vi "K2602 setImeasV.vi"(8 "Settings":T1={"Channel"=enum."Channel A", "Vset"=1e-05, "NPLC"=1.0, "I compliance"=3.0, "Repeat time"=3, "Delay ms"=10.0, "4-wire"=FALSE}, 11 "SMU":refnum<visa-resource-name>="GPIB0::26::INSTR") -> (0 "error out":errorcluster, 1 "Vavg":dbl=0.09425289999999999, 2 "Imeas":dbl[](array[numeric])=[1e-05, 1e-05, 1e-05], 3 "Vmeas":dbl[](array[numeric])=[0.0943061, 0.0942282, 0.0942244])   [LabVIEW 2012]
uses:
  SMU Settings.ctl
  <instrlib>/KE26XX/KE26XX.lvlib
  <vilib>/Analysis/NI_AALBase.lvlib
panel:
  out "Final Script":string="smu = smua\r\nsmusense = smu.SENSE_LOCAL\r\niset = 1.000000E-5\r\nnplc = 1.000000E+0\r\nvlimit = 3.000000E+0\r\nreptime = 3\r\ndelaytime = 1.000000E-2\r\nsmu.reset()\nsmu.source.func = smu.OUTPUT_DCAMPS\nsmu.measure.autozero\t= smu.AUTOZERO_ONCE\nsmu.measure.autorangev\t= smu.AUTORANGE_ON\nsmu.source.autorangei\t= smu.AUTORANGE_ON\nsmu.sense = smusense\n\nsmu.source.leveli = iset\nsmu.source.limitv = vlimit\nsmu.measure.nplc = nplc \n\n-- Setup a buffer to store the result(s) in and start testing.\nsmu.nvbuffer1.clear()\nsmu.nvbuffer1.appendmode = 1\nsmu.nvbuffer1.collecttimestamps = 1\nsmu.nvbuffer1.collectsourcevalues = 1\nsmu.source.output = smu.OUTPUT_ON\n\nfor j = 1,reptime do\n    smu.source.leveli = iset\n    if j == 1 then\n        delay(0.01)  \n    end\n\t   delay(delaytime)                  -- Wait desired settling time.\n    smu.measure.v(smu.nvbuffer1)  -- Measure voltage and store in reading buffer.\nend\nsmu.source.output = smu.OUTPUT_OFF"
  in  "Vmeas Script":string="smu.reset()\nsmu.source.func = smu.OUTPUT_DCAMPS\nsmu.measure.autozero\t= smu.AUTOZERO_ONCE\nsmu.measure.autorangev\t= smu.AUTORANGE_ON\nsmu.source.autorangei\t= smu.AUTORANGE_ON\nsmu.sense = smusense\n\nsmu.source.leveli = iset\nsmu.source.limitv = vlimit\nsmu.measure.nplc = nplc \n\n-- Setup a buffer to store the result(s) in and start testing.\nsmu.nvbuffer1.clear()\nsmu.nvbuffer1.appendmode = 1\nsmu.nvbuffer1.collecttimestamps = 1\nsmu.nvbuffer1.collectsourcevalues = 1\nsmu.source.output = smu.OUTPUT_ON\n\nfor j = 1,reptime do\n    smu.source.leveli = iset\n    if j == 1 then\n        delay(0.01)  \n    end\n\t   delay(delaytime)                  -- Wait desired settling time.\n    smu.measure.v(smu.nvbuffer1)  -- Measure voltage and store in reading buffer.\nend\nsmu.source.output = smu.OUTPUT_OFF"
  in  "Read Points":u32=50
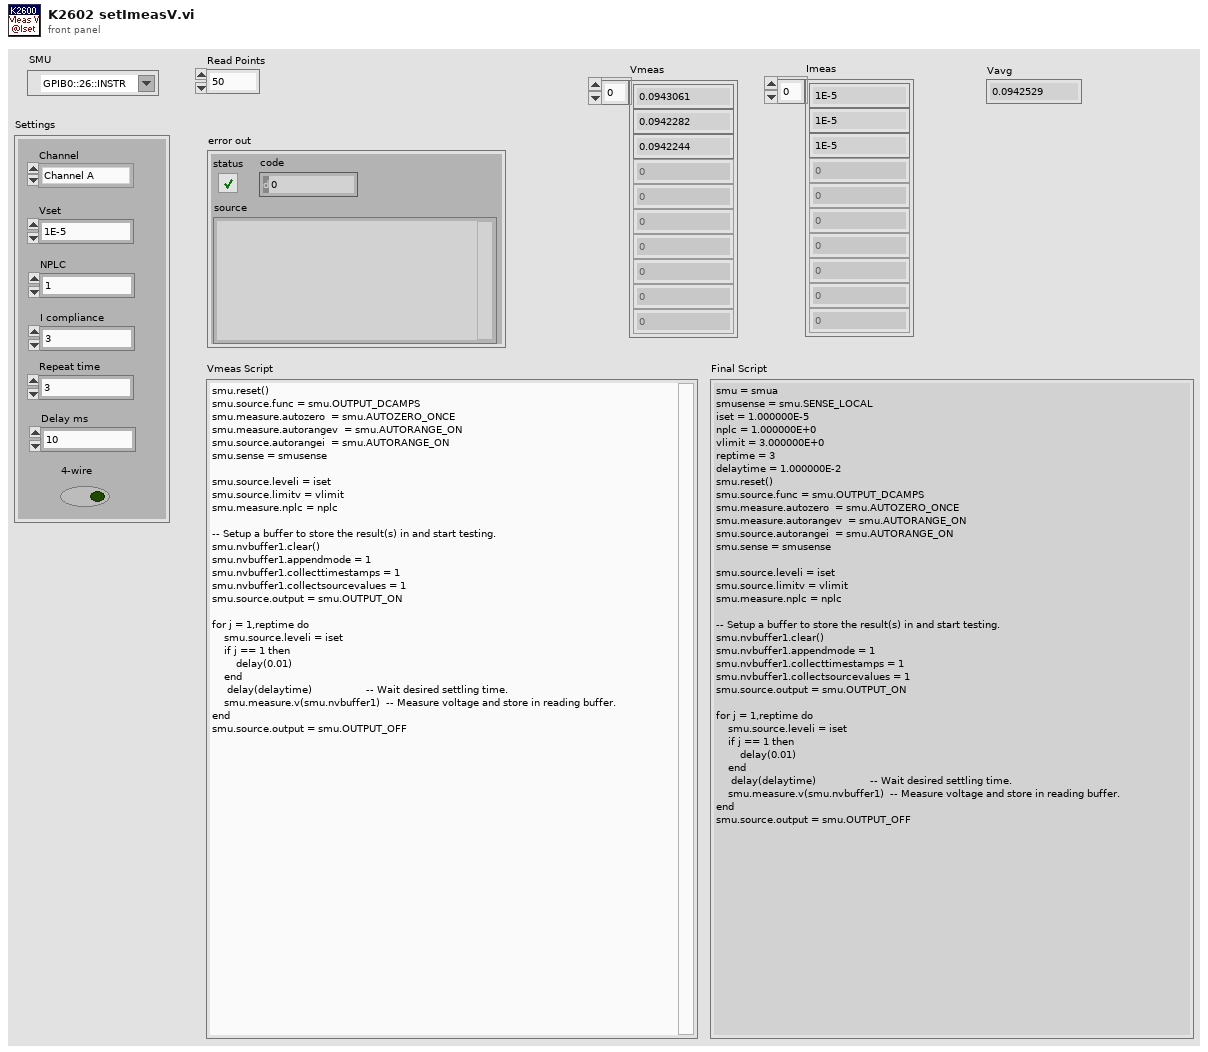
[diagram p1: front panel]
types:
  T1 = typedef "SMU Settings.ctl" = cluster{"Channel":enum32{"Channel A", "Channel B"}, "Vset":dbl, "NPLC":dbl, "I compliance":dbl, "Repeat time":u16, "Delay ms":dbl, "4-wire":bool}
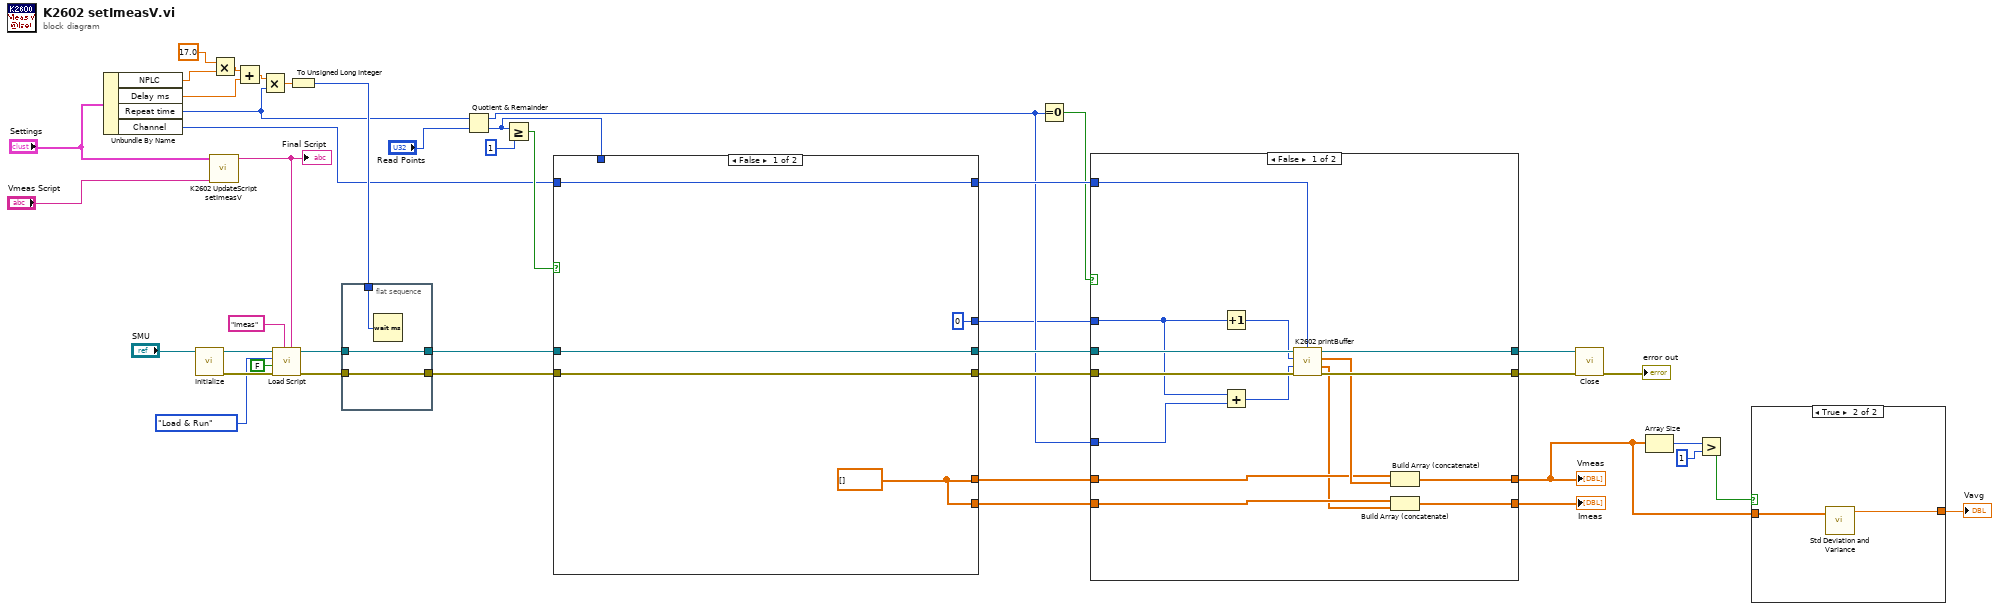
[diagram p0: block diagram]
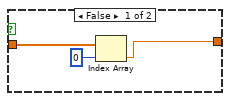
[diagram p2: hidden frame]
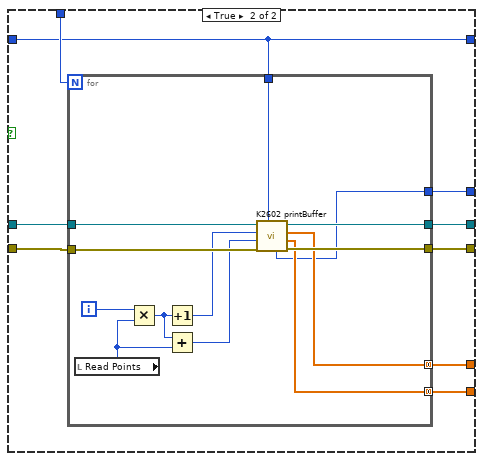
[diagram p4: hidden frame]
diagram:
  n1 = Unbundle By Name("Settings") -> ("NPLC"=w35:dbl, "Delay ms"=w4:dbl, "Repeat time"=w2:u16, "Channel"=w26:enum32{"Channel A", "Channel B"})
  n2 = call <instrlib>:"Initialize.vi"("VISA resource name"="SMU") -> ("error out"=w41:errorcluster, "VISA resource name out"=w42:refnum<visa-resource-name>)  [unwired: 9 in]
  n3 = call "K2602 UpdateScript setImeasV.vi"("Script"="Vmeas Script", "Settings"="Settings") -> ("Output"=w32:string)  [unwired: 9 in]
  "Final Script" <- w32
  n4 = Multiply(x=17.0, y=w35) -> (x*y=w5:dbl)
  n5 = Add(x=w5, y=w4) -> (x+y=w3:dbl)
  n6 = Multiply(x=w3, y=w2) -> (x*y=w1:dbl)
  n7 = call <instrlib>:"Load Script.vi"("Script"=w32, "Script Name"="Imeas", "error in"=w41, "Save (No)"=FALSE, "Load Options (Load)"=enum16{"Load", "Load & Run"}."Load & Run", "VISA resource name"=w42) -> ("error out"=w30:errorcluster, "VISA resource name out"=w31:refnum<visa-resource-name>)  [unwired: 4 out]
  n8 = To Unsigned Long Integer(number=w1) -> (unsigned 32bit integer=w33:u32)
  n9 = flat-sequence {
    tunnel: w33 -> [w46]
    tunnel: w31 -> [w45]
    tunnel: [w45] -> w24
    tunnel: w30 -> [w44]
    tunnel: [w44] -> w23
    frame #0 {
      n10 = Wait (ms)(milliseconds to wait=w46) -> ()  [unwired: 1 out]
    }
  }
  n11 = Quotient & Remainder(x=w2, y="Read Points") -> (x-y*floor(x/y)=w13:u32, floor(x/y)=w25:u32)
  n12 = Greater Or Equal?(x=w25, y=u32 1) -> (x >= y?=w27:bool)
  n13 = case shown="False" w27 {
    tunnel: w26 -> [w51 w55]
    tunnel: [w51 w55] -> w22
    tunnel: w25 -> [_ w60]
    tunnel: w24 -> [w50 w59]
    tunnel: w23 -> [w49 w58]
    tunnel: [w50 w57] -> w19
    tunnel: [w49 w56] -> w18
    tunnel: [w48 w54] -> w21
    tunnel: [w48 w53] -> w20
    tunnel: [u32 0 ("End Index out") w52] -> w11
    frame False {
      w48 = dbl[] [] ("array type (2D Dbl)")
    }
    frame True {
      n14 = for {
        N: w60 -> [_]
        tunnel: w59 -> [w73]
        tunnel: w58 -> [w72]
        tunnel: [w71] -> w57
        tunnel: [w70] -> w56
        tunnel: w55 -> [w69]
        tunnel: [w63] -> w54 mode=concatenating
        tunnel: [w62] -> w53 mode=concatenating
        tunnel: [w61] -> w52
        i -> [w68]
        n15 = local read "Read Points"() -> (w66:u32)
        n16 = Multiply(x=w68, y=w66) -> (x*y=w67:u32)
        n17 = Increment(x=w67) -> (x+1=w65:u32)
        n18 = Add(x=w67, y=w66) -> (x+y=w64:u32)
        n19 = call "K2602 printBuffer.vi"("Channel"=w69, "error in (no error)"=w72, "End Index"=w64, "Start Index"=w65, "SMU"=w73) -> ("error out"=w70:errorcluster, "V array"=w62:dbl[], "I array"=w63:dbl[], "SMU out"=w71:refnum<visa-resource-name>, "End Index out"=w61:u32)  [unwired: 2 in]
      }
    }
  }
  n20 = Equal To 0?(x=w13) -> (x = 0?=w12:bool)
  n21 = case shown="False" w12 {
    tunnel: w22 -> [w84 _]
    tunnel: w21 -> [w78 w90]
    tunnel: w20 -> [w76 w89]
    tunnel: w19 -> [w88 w92]
    tunnel: w18 -> [w87 w91]
    tunnel: [w86 w92] -> w17
    tunnel: [w85 w91] -> w16
    tunnel: [w77 w90] -> w7
    tunnel: [w74 w89] -> w15
    tunnel: w13 -> [w81 _]
    tunnel: w11 -> [w82 _]
    frame False {
      n22 = Increment(x=w82) -> (x+1=w83:u32)
      n23 = Add(x=w82, y=w81) -> (x+y=w80:u32)
      n24 = call "K2602 printBuffer.vi"("Channel"=w84, "error in (no error)"=w87, "End Index"=w80, "Start Index"=w83, "SMU"=w88) -> ("error out"=w85:errorcluster, "V array"=w75:dbl[], "I array"=w79:dbl[], "SMU out"=w86:refnum<visa-resource-name>)  [unwired: 2 in, 1 out]
      n25 = Build Array (concatenate)(w78, w79) -> (w77:dbl[])
      n26 = Build Array (concatenate)(w76, w75) -> (w74:dbl[])
    }
    frame True {
    }
  }
  "Vmeas" <- w7
  "Imeas" <- w15
  n27 = call <instrlib>:"Close.vi"("error in (no error)"=w16, "VISA resource name"=w17) -> ("error out"=→"error out":errorcluster)  [unwired: 9 in]
  n28 = Array Size(array=w7) -> (size(s)=w10:i32)
  n29 = Greater?(x=w10, y=1) -> (0:w8:bool)
  n30 = case shown="True" w8 {
    tunnel: w7 -> [w95 w97]
    tunnel: [w93 w96] -> w6
    frame False {
      n31 = Index Array(array=w95, index=0) -> (element=w93:dbl)
    }
    frame True {
      n32 = call <vilib>:"Std Deviation and Variance.vi"("X"=w97) -> ("mean"=w96:dbl)  [unwired: 1 in, 2 out]
    }
  }
  "Vavg" <- w6
